vi "Func_Glob_Psi_k_PN.vi"(4 "Action":enum16{"Read", "Write"}(ring), 5 "k2 coeffs IN":T1 {"x locations" format="%.4g"; "coefficients" format="%.4g"}, 6 "k1 coeffs IN":T1 {"x locations" format="%.4g"; "coefficients" format="%.4g"}, 7 "Psi2 coeffs IN":T1 {"x locations" format="%.4g"; "coefficients" format="%.4g"}, 8 "Psi1 coeffs IN":T1 {"x locations" format="%.4g"; "coefficients" format="%.4g"}) -> (0 "k2 coeffs OUT":T1 {"x locations" format="%.4g"; "coefficients" format="%.4g"}, 1 "k1 coeffs OUT":T1 {"x locations" format="%.4g"; "coefficients" format="%.4g"}, 2 "Psi2 coeffs OUT":T1 {"x locations" format="%.4g"; "coefficients" format="%.4g"}, 3 "Psi1 coeffs OUT":T1 {"x locations" format="%.4g"; "coefficients" format="%.4g"})   [LabVIEW 2011]
uses:
  <vilib>/gmath/interp.llb/in_piecewise interp poly control.ctl
  <vilib>/gmath/NI_Gmath.lvlib
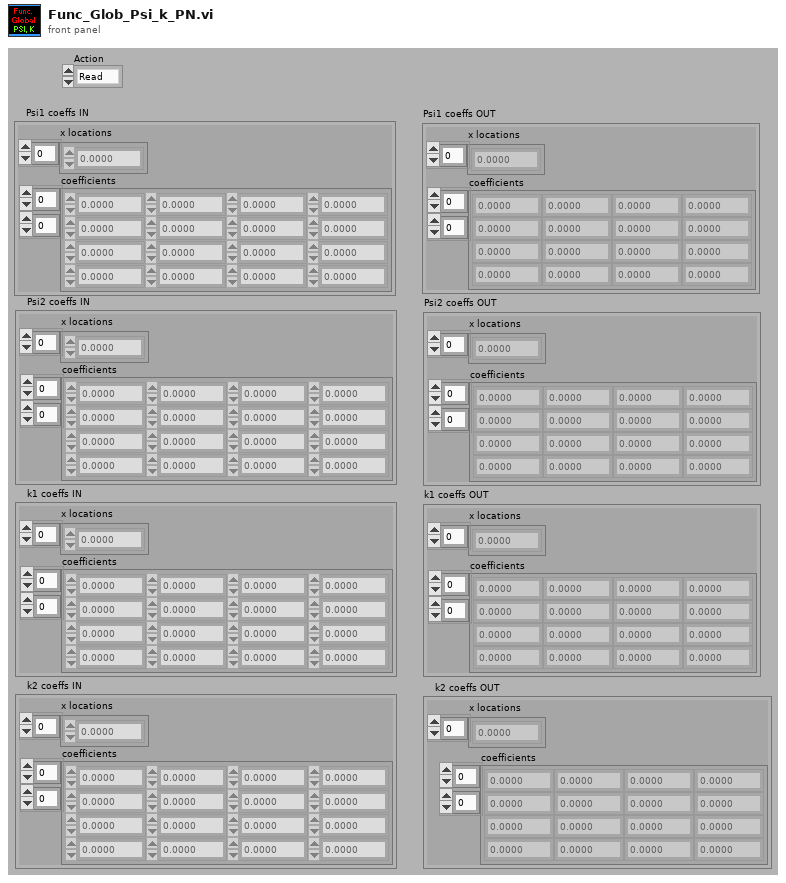
[diagram p1: front panel]
types:
  T1 = typedef "NI_Gmath.lvlib/in_piecewise interp poly control.ctl" = cluster{"x locations":dbl[], "coefficients":dbl[][]}
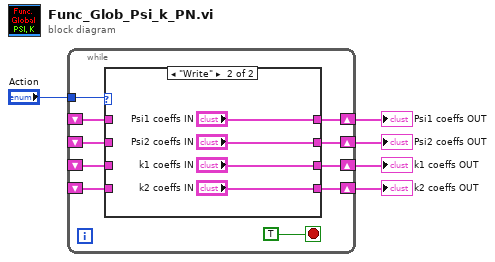
[diagram p0: block diagram]
diagram:
  n1 = while {
    shift-right: [w11] -> w4
    shift-left: _ -> [w13]
    shift-right: [w10] -> w3
    shift-left: _ -> [w12]
    tunnel: "Action" -> [w15]
    shift-right: [w6] -> w1
    shift-left: _ -> [w8]
    shift-right: [w7] -> w2
    shift-left: _ -> [w9]
    stop <- TRUE stop-if-true
    n2 = case shown="\"Write\"" w15 {
      tunnel: w13 -> [w19 _]
      tunnel: w12 -> [w18 _]
      tunnel: [w19 "Psi1 coeffs IN"] -> w11
      tunnel: [w18 "Psi2 coeffs IN"] -> w10
      tunnel: w9 -> [w17 _]
      tunnel: w8 -> [w16 _]
      tunnel: [w17 "k1 coeffs IN"] -> w7
      tunnel: [w16 "k2 coeffs IN"] -> w6
      frame "Read" {
      }
      frame "Write" {
      }
    }
  }
  "Psi1 coeffs OUT" <- w4
  "Psi2 coeffs OUT" <- w3
  "k1 coeffs OUT" <- w2
  "k2 coeffs OUT" <- w1
